vi "Event - 1000 msec DVR.vi"() -> ()   [LabVIEW 2011]
doc: "This VI calls a DVR Timer and resets the timer every 1000 msec. The purpose is to demonstrate using multiple instances of an object in a LabVIEW application.\n\nAAL 9/09"
panel:
  out "Elapsed Time (ms)":u32
  in  "Exit":bool
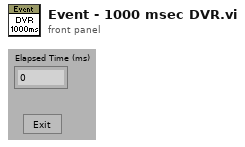
[diagram p1: front panel]
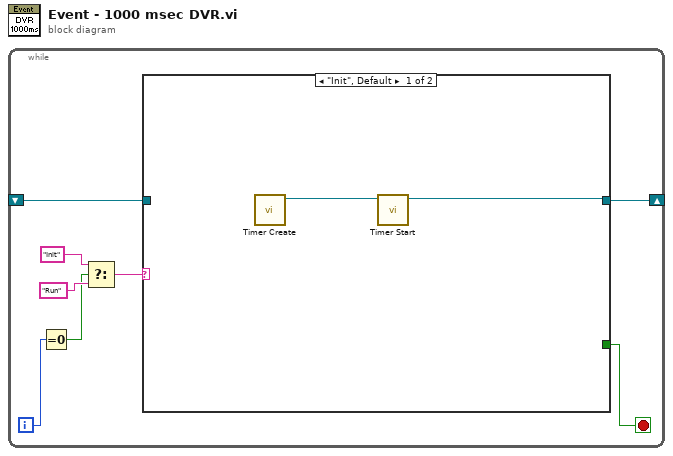
[diagram p0: block diagram]
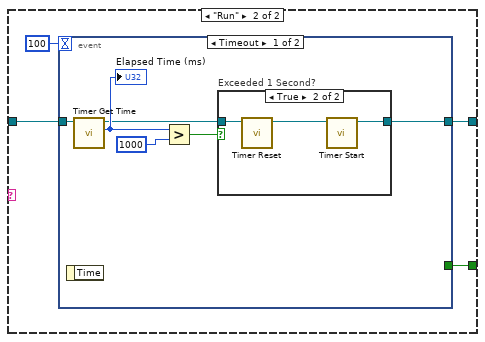
[diagram p2: hidden frame]
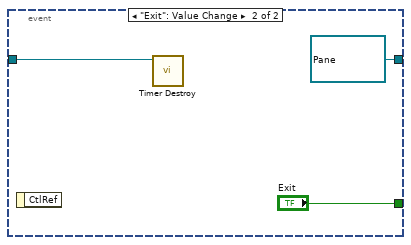
[diagram p4: hidden frame]
diagram:
  n1 = while {
    shift-right: [w2] -> _
    shift-left: _ -> [w1]
    i -> [w7]
    stop <- w8 stop-if-true
    n2 = Equal To 0?(x=w7) -> (x = 0?=w5:bool)
    n3 = Select(t="Init", s=w5, f="Run") -> (s? t:f=w3:string)
    n4 = case shown="\"Init\", Default" w3 {
      tunnel: [_ w13] -> w8
      tunnel: [w9 w11] -> w2
      tunnel: w1 -> [_ w12]
      frame "Init", Default {
        n5 = call "Timer Create.vi"() -> ("Timer reference out"=w10:refnum<data-value>)  [unwired: 10 in, 1 out]
        n6 = call "Timer Start.vi"("Timer reference"=w10) -> ("Timer reference  out"=w9:refnum<data-value>)  [unwired: 9 in, 1 out]
      }
      frame "Run" {
        n7 = event shown="[0] Timeout" {
          selector: _ -> [_ _]
          dyn-events: _ -> [_ _]
          timeout: 100 -> [_ _]
          tunnel: [_ "Exit"] -> w13
          tunnel: w12 -> [w20 w26]
          tunnel: [w15 refnum<data-value> refnum ("Timer reference  out")] -> w11
          event Timeout {
            n8 = event-data() -> ()  [unwired: 1 in, 1 out]
            n9 = call "Timer Get Time.vi"("Timer reference"=w20) -> ("Elapsed Time (ms)"=w19:u32, "Timer reference  out"=w16:refnum<data-value>)  [unwired: 7 in, 2 out]
            "Elapsed Time (ms)" <- w19
            n10 = Greater?(x=w19, y=u32 1000) -> (0:w17:bool)
            n11 = case "Exceeded 1 Second?" shown="True" w17 {
              tunnel: w16 -> [w21 w24]
              tunnel: [w21 w22] -> w15
              frame False {
              }
              frame True {
                n12 = call "Timer Reset.vi"("Timer reference"=w24) -> ("Timer reference  out"=w23:refnum<data-value>)  [unwired: 9 in, 1 out]
                n13 = call "Timer Start.vi"("Timer reference"=w23) -> ("Timer reference  out"=w22:refnum<data-value>)  [unwired: 9 in, 1 out]
              }
            }
          }
          event "Exit": Value Change {
            n14 = event-data() -> ()  [unwired: 1 in, 1 out]
            n15 = call "Timer Destroy.vi"("Timer reference"=w26) -> ()  [unwired: 10 in, 1 out]
          }
        }
      }
    }
  }
